vi "Execute.vi"(8 "Error In":errorcluster, 9 "Workspace":T1, 10 "Control In":T2={"I-O.lvclass"=refnum, "Gantry"=refnum, "Dispenser"="COM1"}, 11 "Dispense in":refnum<class "Dispense.lvclass">) -> (0 "Error Out":errorcluster, 2 "Control Out":T2={"I-O.lvclass"=refnum, "Gantry"=refnum, "Dispenser"="COM1"}, 3 "Dispense out":refnum<class "Dispense.lvclass">)   [LabVIEW 2018, in "Dispense.lvclass"]
uses:
  Dispense.lvclass
  Controller/Controllers.ctl
  Controller/I-O/I-O.lvclass
  C:/Program Files (x86)/Aerotech/A3200/LabVIEW/2010/Bin/Aerotech.A3200.dll
  Program Files (x86)/Aerotech/A3200/LabVIEW/2010/Bin/Aerotech.A3200.dll
  Workspace/Workspace.ctl
  Dispense.lvclass/Dispense.ctl
  Controller/Controller.lvclass
  Workspace/Fixture.lvclass
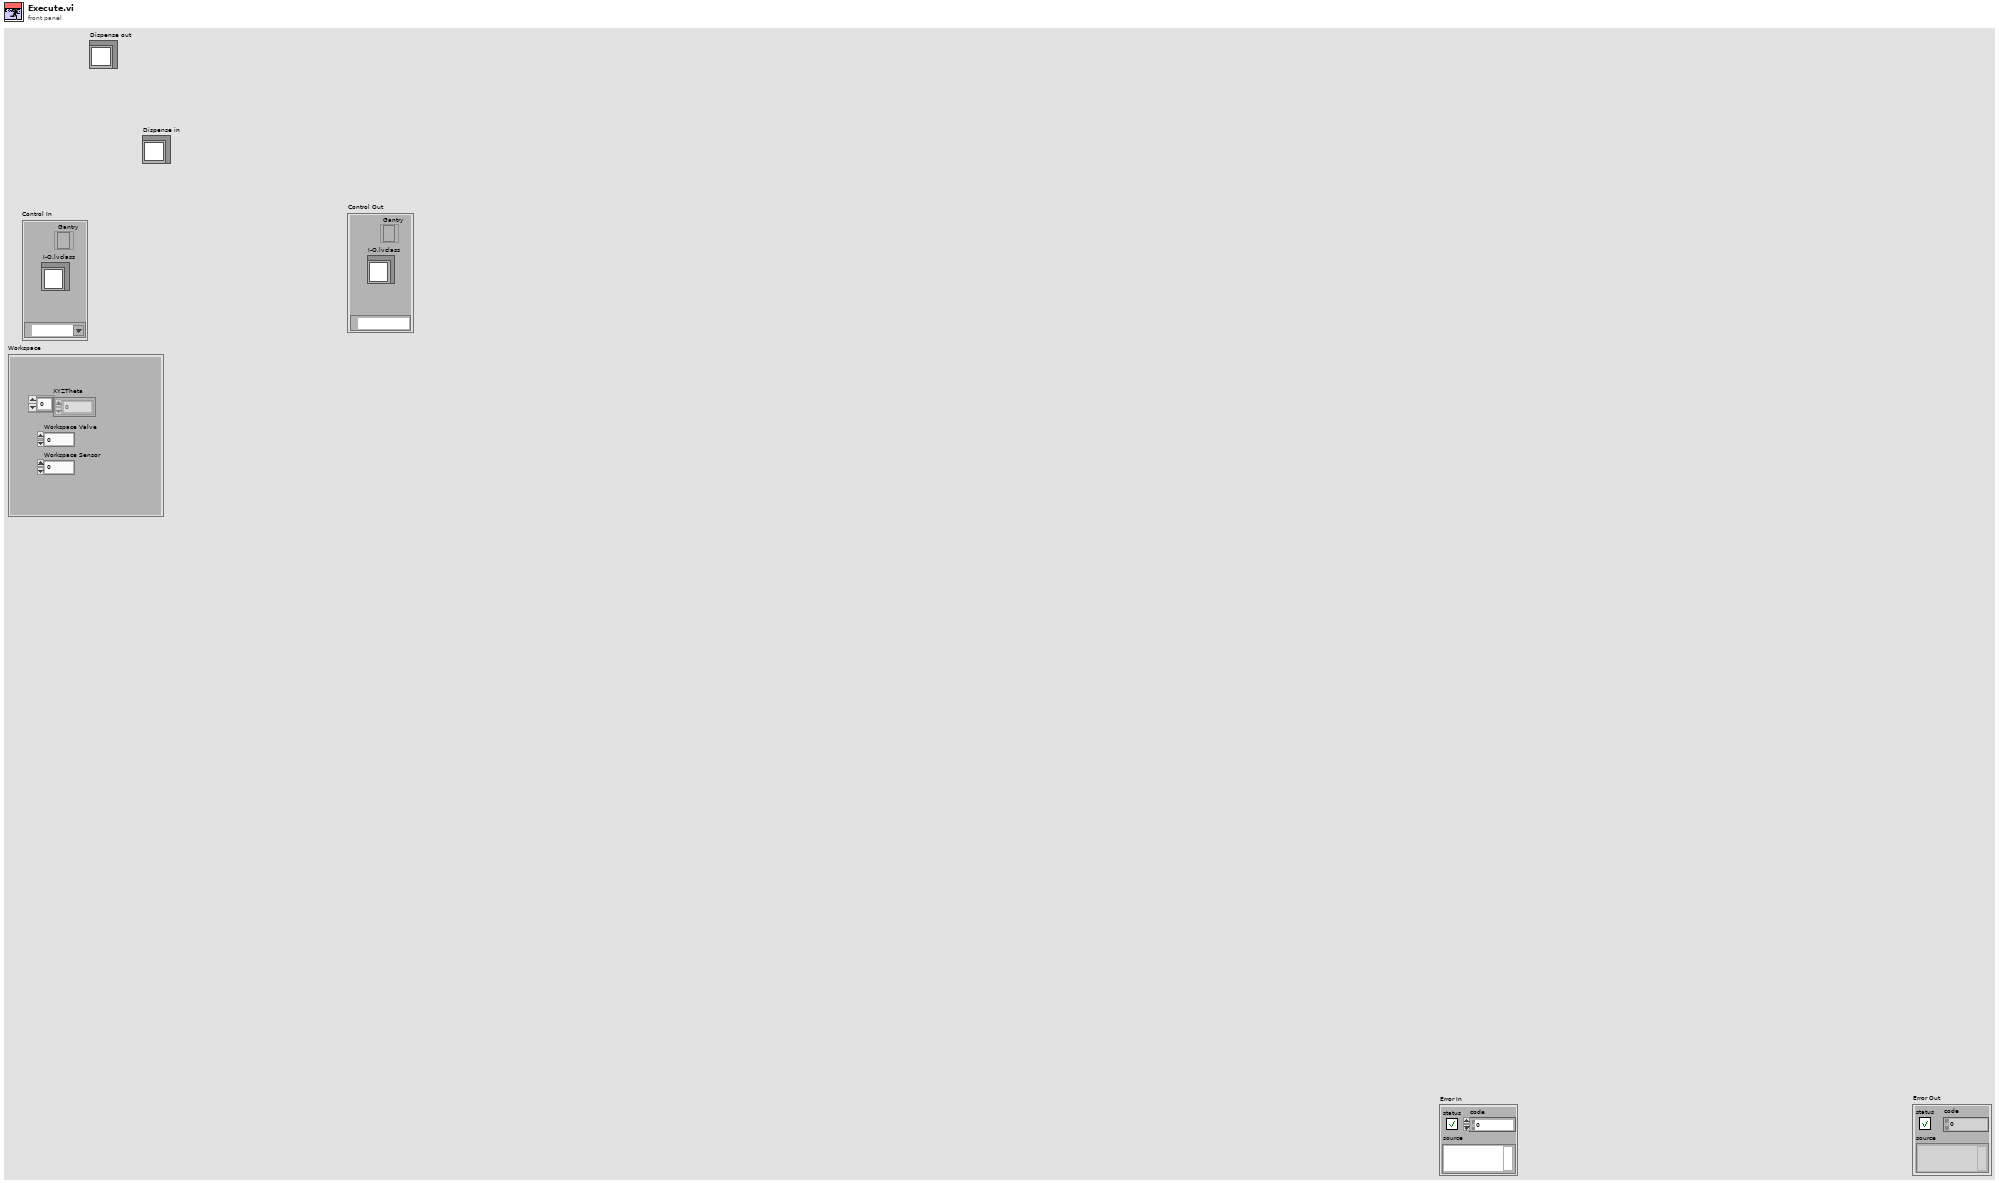
[diagram p1: front panel]
types:
  T1 = typedef "Fixture.lvclass/Workspace.ctl" = cluster{"XYZTheta":dbl[], "Workspace Valve":i32, "Workspace Sensor":i32}
  T2 = typedef "Controller.lvclass/Controllers.ctl" = cluster{"I-O.lvclass":refnum<class "I-O.lvclass">, "Gantry":refnum<k24>, "Dispenser":refnum<visa-resource-name>}
  T3 = cluster{"Time to Go Down":i32, "Time to Dispense":i32}[]
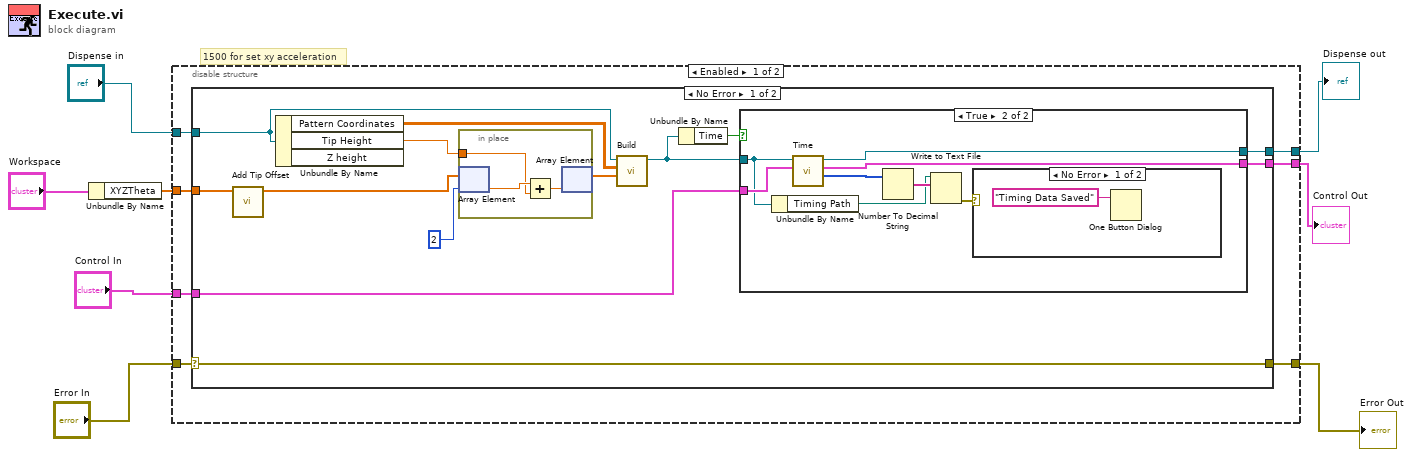
[diagram p0: block diagram]
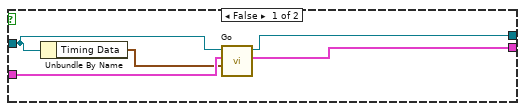
[diagram p2: hidden frame]
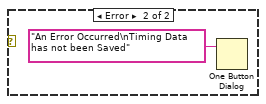
[diagram p3: hidden frame]
diagram:
  # "1500 for set xy acceleration"
  n1 = Unbundle By Name("Workspace") -> ("XYZTheta"=w2:dbl[])
  n2 = disable-structure shown="Enabled" {
    disable-tunnel: "Control In" -> [w15 w50]
    disable-tunnel: [w14 w50] -> w7
    disable-tunnel: "Dispense in" -> [w13 w52]
    disable-tunnel: "Error In" -> [w12 w51]
    disable-tunnel: [w11 w51] -> w4
    disable-tunnel: w2 -> [w10 _]
    disable-tunnel: [w9 w52] -> w1
    frame Enabled {
      n3 = case shown="No Error" w12 {
        selector: w12 -> [w28 w48]
        tunnel: w15 -> [w18 w49]
        tunnel: [w17 w49] -> w14
        tunnel: w13 -> [w21 w47]
        tunnel: [w28 w48] -> w11
        tunnel: w10 -> [w16 _]
        tunnel: [w26 w47] -> w9
        frame No Error {
          n4 = call "Add Tip Offset.vi"("XYZTheta"=w16) -> ("XYZTheta"=w20:dbl[])  [unwired: 10 in]
          n5 = Unbundle By Name(w21) -> ("Pattern Coordinates"=w25:dbl[][], "Tip Height"=w22:dbl)  [unwired: 1 out]
          n6 = in-place {
            in-place-border: w22 -> [w44]
            n7 = in-place-array #1(w20, 2) -> (w46:dbl)
            n8 = Add(x=w46, y=w44) -> (x+y=w45:dbl)
            n9 = in-place-array #1(w45) -> (w23:dbl[])  [unwired: 1 out]
          }
          n10 = call-dynamic "Build.vi"("XYZTheta"=w23, "Pattern Coordinates"=w25, "Dispense in"=w21) -> ("Dispense out"=w27:refnum<class "Dispense.lvclass">)  [unwired: 8 in]
          n11 = Unbundle By Name(w27) -> ("Time"=w19:bool)
          n12 = case shown="True" w19 {
            tunnel: w27 -> [w33 w35]
            tunnel: w18 -> [w32 w37]
            tunnel: [w29 w36] -> w17
            tunnel: [w30 w34] -> w26
            frame False {
              n13 = Unbundle By Name(w33) -> ("Timing Data"=w31:T3)
              n14 = call-dynamic "Go.vi"("Timing Data"=w31, "Control In"=w32, "Dispense in"=w33) -> ("Control Out"=w29:T2, "Dispense Out"=w30:refnum<class "Dispense.lvclass">)  [unwired: 7 in]
            }
            frame True {
              n15 = Unbundle By Name(w35) -> ("Timing Path"=w39:path)
              n16 = call-dynamic "Time.vi"("Control In"=w37, "Dispense in"=w35) -> ("Timing Data"=w38:i32[], "Control Out"=w36:T2, "Dispense out"=w34:refnum<class "Dispense.lvclass">)  [unwired: 6 in, 1 out]
              n17 = Number To Decimal String(number=w38) -> (decimal integer string=w40:string[])  [unwired: 1 in]
              n18 = Write to Text File(file (use dialog)=w39, text=w40) -> (error out=w41:errorcluster)  [unwired: 2 in, 2 out]
              n19 = case shown="No Error" w41 {
                frame No Error {
                  n20 = One Button Dialog(message="Timing Data Saved") -> ()  [unwired: 1 in, 1 out]
                }
                frame Error {
                  n21 = One Button Dialog(message="An Error Occurred\nTiming Data has not been Saved") -> ()  [unwired: 1 in, 1 out]
                }
              }
            }
          }
        }
        frame Error {
        }
      }
    }
    frame Disabled {
    }
  }
  "Control Out" <- w7
  "Error Out" <- w4
  "Dispense out" <- w1
